vi "Phase9225-7_FPGA.vi"(3 "dT [s]":fxp<+/-,36,-5>, 4 "Frequency [Hz]":fxp<+,36,7>, 5 "dBin [-0.5,0.5)":fxp<+/-,36,0>, 6 "phase(i) [pi rad]":fxp<+/-,36,2>) -> (1 "Phase [rad]":fxp<+/-,36,3>)   [LabVIEW 2021]
uses:
  <vilib>/rvi/FXPMathLib/FxpInterpret/XNode/nifxpmath_Interpret.xnode
  <vilib>/rvi/FXPMathLib/FxpSub/XNode/nifxpmath_Sub.xnode
  <vilib>/rvi/FXPMathLib/sim/FxpSim.dll
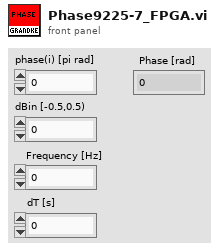
[diagram p1: front panel]
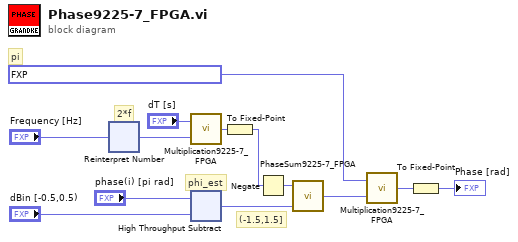
[diagram p0: block diagram]
diagram:
  # "(-1.5,1.5]"
  # "pi"
  # "2*f"
  # "phi_est"
  n1 = xnode "Reinterpret Number"("x"="Frequency [Hz]") -> ("y"=w6:fxp<+,36,8>)
  n2 = call "Multiplication9225-7_FPGA.vi"("y <+/-44,8>"=w6, "x <+/-47,6>"="dT [s]") -> ("x*y <+/-49,13>"=w11:fxp<+/-,49,13>)
  n3 = xnode "High Throughput Subtract"("x"="phase(i) [pi rad]", "y"="dBin [-0.5,0.5)") -> ("x-y"=w4:fxp<+/-,36,2>)
  n4 = To Fixed-Point(number=w11) -> (fixed-point=w3:fxp<+/-,36,2>)  [unwired: 1 in]
  n5 = Negate(x=w3) -> (-x=w5:fxp<+/-,36,2>)
  n6 = call "PhaseSum9225-7_FPGA.vi"("phi2 [pi rad]"=w4, "phi1 [pi rad]"=w5) -> ("phi1+phi2 [pi rad] (-1,1]"=w2:fxp<+/-,36,2>)  [unwired: 3 in]
  n7 = call "Multiplication9225-7_FPGA.vi"("y <+/-44,8>"=w2, "x <+/-47,6>"=fxp<+,36,2> 3.1415926535846666 ("x")) -> ("x*y <+/-49,13>"=w12:fxp<+/-,49,13>)
  n8 = To Fixed-Point(number=w12) -> (fixed-point=→"Phase [rad]":fxp<+/-,36,3>)  [unwired: 1 in]
